vi "SWING_turn_left.vi"() -> ()   [LabVIEW 2015]
uses:
  <vilib>/NXT/Subs/MotorOutput.ctl
  <vilib>/NXT/Block Support/NXT_InputPort.ctl
  <vilib>/NXT/NXTIO Xnodes/NXTIONodeSubVIs/LEGOStopAllMotors.vi
  <vilib>/NXT/Dual Mode Library/Waits/Wait_Num.vi
  <vilib>/NXT/Dual Mode Library/Motors/MotorReverse.vi
  <vilib>/NXT/Dual Mode Library/Motors/MotorOn.vi
  <vilib>/NXT/Dual Mode Library/Sensors/Light_On.vi
  <vilib>/NXT/Dual Mode Library/Sensors/Sonar_cm.vi
  <vilib>/NXT/Dual Mode Library/Motors/MotorCoast.vi
  <vilib>/NXT/Subs/LVHSConnector.ctl
  <vilib>/NXT/NXTIO Xnodes/NXTIOXNode/NXTIO.xnode
  <vilib>/NXT/LegoClasses/BrickReference/BrickReference.lvclass
panel:
  in  "stop":bool
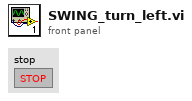
[diagram p1: front panel]
types:
  T1 = typedef "MotorOutput.ctl" = u8
  T2 = typedef "LVHSConnector.ctl" = refnum<class "BrickReference.lvclass">
  T3 = typedef "NXT_InputPort.ctl" = u32
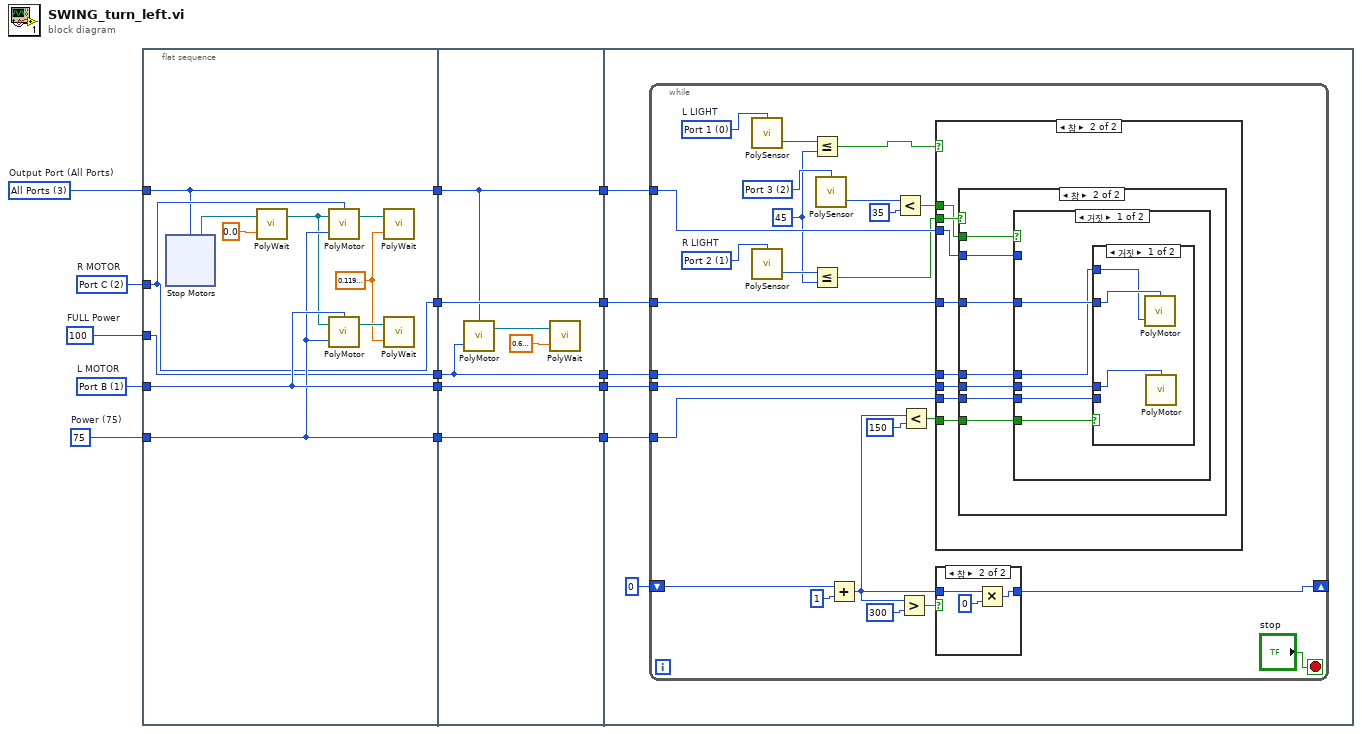
[diagram p0: block diagram]
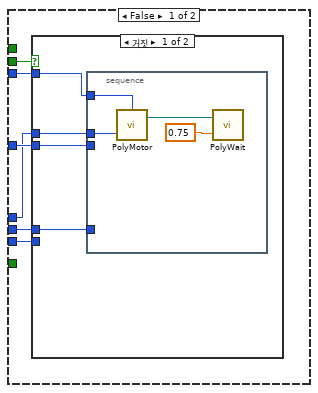
[diagram p3: hidden frame]
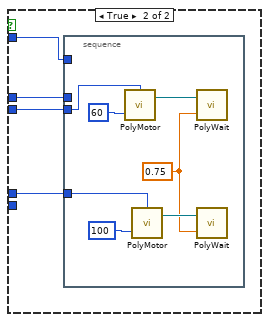
[diagram p4: hidden frame]
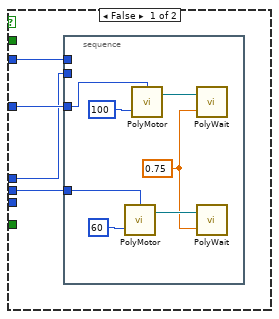
[diagram p5: hidden frame]
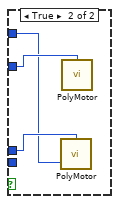
[diagram p6: hidden frame]
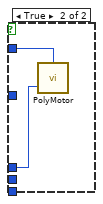
[diagram p7: hidden frame]
diagram:
  w11 = 100  # FULL Power
  w12 = 75  # Power (75)
  w13 = T1 2 items=["Port A"=0, "Port B"=1, "Port C"=2, "Ports A & B"=4, "Ports A & C"=5, "Ports B & C"=6, "All Ports"=3]  # R MOTOR
  w14 = T1 1 items=["Port A"=0, "Port B"=1, "Port C"=2, "Ports A & B"=4, "Ports A & C"=5, "Ports B & C"=6, "All Ports"=3]  # L MOTOR
  w15 = T1 3 items=["Port A"=0, "Port B"=1, "Port C"=2, "Ports A & B"=4, "Ports A & C"=5, "Ports B & C"=6, "All Ports"=3]  # Output Port (All Ports)
  n1 = flat-sequence {
    tunnel: w15 -> [w20]
    tunnel: w14 -> [w26]
    tunnel: w13 -> [w24]
    tunnel: w12 -> [w25]
    tunnel: w11 -> [w16]
    tunnel: [w20] -> w10
    tunnel: [w26] -> w8
    tunnel: [w24] -> w6
    tunnel: [w25] -> w4
    tunnel: [w16] -> w2
    tunnel: w10 -> [w34]
    tunnel: [w34] -> w9
    tunnel: w8 -> [w38]
    tunnel: [w38] -> w7
    tunnel: w6 -> [w37]
    tunnel: [w37] -> w5
    tunnel: w4 -> [w36]
    tunnel: [w36] -> w3
    tunnel: w2 -> [w35]
    tunnel: [w35] -> w1
    tunnel: w9 -> [w44]
    tunnel: w7 -> [w43]
    tunnel: w5 -> [w42]
    tunnel: w3 -> [w41]
    tunnel: w1 -> [w40]
    frame #0 {
      w21 = sgl 0.12 ("Time (1 sec)")
      n2 = xnode "Stop Motors"("Motors"=w20) -> ("NXT/EV3"=w19:T2)  [unwired: 1 in]
      n3 = call-poly <vilib>:"PolyWait.vi"("Time (1 sec)"=sgl 0.0, "NXT/EV3"=w19) -> ("NXT/EV3"=w18:T2)  [unwired: 2 in]
      n4 = call-poly <vilib>:"PolyMotor.vi"("Power (75)"=w25, "NXT/EV3"=w18, "Output Port (All Ports)"=w24) -> ("NXT/EV3"=w22:T2)  [unwired: 1 out]
      n5 = call-poly <vilib>:"PolyMotor.vi"("Power (75)"=w25, "NXT/EV3"=w18, "Output Port (All Ports)"=w26) -> ("NXT/EV3"=w23:T2)  [unwired: 1 out]
      n6 = call-poly <vilib>:"PolyWait.vi"("Time (1 sec)"=w21, "NXT/EV3"=w22) -> ()  [unwired: 2 in, 1 out]
      n7 = call-poly <vilib>:"PolyWait.vi"("Time (1 sec)"=w21, "NXT/EV3"=w23) -> ()  [unwired: 2 in, 1 out]
    }
    frame #1 {
      n8 = call-poly <vilib>:"PolyMotor.vi"("Power (75)"=w35, "Output Port (All Ports)"=w34) -> ("NXT/EV3"=w33:T2)  [unwired: 1 in, 1 out]
      n9 = call-poly <vilib>:"PolyWait.vi"("Time (1 sec)"=sgl 0.7, "NXT/EV3"=w33) -> ()  [unwired: 2 in, 1 out]
    }
    frame #2 {
      n10 = while {
        tunnel: w44 -> [w64]
        tunnel: w43 -> [w63]
        tunnel: w42 -> [w62]
        tunnel: w41 -> [w61]
        tunnel: w40 -> [w60]
        shift-right: [w50] -> _
        shift-left: i16 0 ("y") -> [w55]
        stop <- "stop" stop-if-true
        w59 = T3 2 items=["Port 1", "Port 2", "Port 3", "Port 4"] ("Port (Port 4)")
        w65 = T3 1 items=["Port 1", "Port 2", "Port 3", "Port 4"]  # R LIGHT
        w68 = T3 0 items=["Port 1", "Port 2", "Port 3", "Port 4"]  # L LIGHT
        w51 = i16 45 ("Scaled Value")
        n11 = call-poly <vilib>:"PolySensor.vi"("Port (Port 3)"=w68) -> ("Scaled Value"=w67:i16)  [unwired: 2 in, 1 out]
        n12 = call-poly <vilib>:"PolySensor.vi"("Port (Port 3)"=w65) -> ("Scaled Value"=w66:i16)  [unwired: 2 in, 1 out]
        n13 = Less Or Equal?(x=w67, y=w51) -> (x <= y?=w46:bool)
        n14 = Less Or Equal?(x=w66, y=w51) -> (x <= y?=w45:bool)
        n15 = call-poly <vilib>:"PolySensor.vi"("Port (Port 4)"=w59) -> ("Distance (cm)"=w58:i16)  [unwired: 2 in, 1 out]
        n16 = Add(x=w55, y=i16 1) -> (x+y=w49:i16)
        n17 = Less?(x=w58, y=i16 35) -> (x < y?=w56:bool)
        n18 = Greater?(x=w49, y=i16 300) -> (0:w54:bool)
        n19 = Less?(x=w49, y=i16 150) -> (x < y?=w47:bool)
        n20 = case shown="참" w46 {
          tunnel: w64 -> [w78 w106]
          tunnel: w61 -> [w77 w105]
          tunnel: w45 -> [w79 w101]
          tunnel: w62 -> [w76 w103]
          tunnel: w63 -> [w75 w104]
          tunnel: w60 -> [w74 w102]
          tunnel: w56 -> [_ w100]
          tunnel: w47 -> [_ w99]
          frame False {
            n21 = case shown="거짓" w79 {
              tunnel: w78 -> [w83 w88]
              tunnel: w77 -> [_ _]
              tunnel: w75 -> [w81 w91]
              tunnel: w76 -> [w80 w90]
              tunnel: w74 -> [w82 w89]
              frame False {
                n22 = stacked-sequence {
                  tunnel: w83 -> [w87]
                  tunnel: w82 -> [w84]
                  tunnel: w81 -> [_]
                  tunnel: w80 -> [_]
                  frame #0 {
                    n23 = call-poly <vilib>:"PolyMotor.vi"("Power (75)"=w84, "Output Port (All Ports)"=w87) -> ("NXT/EV3"=w86:T2)  [unwired: 1 in, 1 out]
                    n24 = call-poly <vilib>:"PolyWait.vi"("Time (1 sec)"=sgl 0.75, "NXT/EV3"=w86) -> ()  [unwired: 2 in, 1 out]
                  }
                }
              }
              frame True {
                n25 = stacked-sequence {
                  tunnel: w91 -> [w94]
                  tunnel: w90 -> [w93]
                  tunnel: w89 -> [_]
                  tunnel: w88 -> [_]
                  frame #0 {
                    w92 = sgl 0.75 ("Time (1 sec)")
                    n26 = call-poly <vilib>:"PolyMotor.vi"("Power (75)"=60 ("Power (75) 5"), "Output Port (All Ports)"=w93) -> ("NXT/EV3"=w95:T2)  [unwired: 1 in, 1 out]
                    n27 = call-poly <vilib>:"PolyMotor.vi"("Power (75)"=100 ("Power (75) 4"), "Output Port (All Ports)"=w94) -> ("NXT/EV3"=w96:T2)  [unwired: 1 in, 1 out]
                    n28 = call-poly <vilib>:"PolyWait.vi"("Time (1 sec)"=w92, "NXT/EV3"=w95) -> ()  [unwired: 2 in, 1 out]
                    n29 = call-poly <vilib>:"PolyWait.vi"("Time (1 sec)"=w92, "NXT/EV3"=w96) -> ()  [unwired: 2 in, 1 out]
                  }
                }
              }
            }
          }
          frame True {
            n30 = case shown="참" w101 {
              tunnel: w106 -> [w108 w124]
              tunnel: w105 -> [_ w121]
              tunnel: w104 -> [w110 w120]
              tunnel: w103 -> [w109 w119]
              tunnel: w102 -> [w107 w123]
              tunnel: w100 -> [_ w122]
              tunnel: w99 -> [_ w118]
              frame False {
                n31 = stacked-sequence {
                  tunnel: w110 -> [w115]
                  tunnel: w109 -> [w111]
                  tunnel: w108 -> [_]
                  tunnel: w107 -> [_]
                  frame #0 {
                    w112 = sgl 0.75 ("Time (1 sec)")
                    n32 = call-poly <vilib>:"PolyMotor.vi"("Power (75)"=60 ("Power (75) 2"), "Output Port (All Ports)"=w115) -> ("NXT/EV3"=w113:T2)  [unwired: 1 in, 1 out]
                    n33 = call-poly <vilib>:"PolyMotor.vi"("Power (75)"=100 ("Power (75) 3"), "Output Port (All Ports)"=w111) -> ("NXT/EV3"=w116:T2)  [unwired: 1 in, 1 out]
                    n34 = call-poly <vilib>:"PolyWait.vi"("Time (1 sec)"=w112, "NXT/EV3"=w116) -> ()  [unwired: 2 in, 1 out]
                    n35 = call-poly <vilib>:"PolyWait.vi"("Time (1 sec)"=w112, "NXT/EV3"=w113) -> ()  [unwired: 2 in, 1 out]
                  }
                }
              }
              frame True {
                n36 = case shown="거짓" w122 {
                  tunnel: w124 -> [_ w137]
                  tunnel: w123 -> [w125 w136]
                  tunnel: w121 -> [w129 _]
                  tunnel: w120 -> [w128 _]
                  tunnel: w119 -> [w127 _]
                  tunnel: w118 -> [w126 _]
                  frame False {
                    n37 = case shown="거짓" w126 {
                      tunnel: w129 -> [_ _]
                      tunnel: w128 -> [w132 w135]
                      tunnel: w127 -> [w131 w134]
                      tunnel: w125 -> [w130 w133]
                      frame False {
                        n38 = call-poly <vilib>:"PolyMotor.vi"("Power (75)"=w130, "Output Port (All Ports)"=w131) -> ()  [unwired: 1 in, 2 out]
                        n39 = call-poly <vilib>:"PolyMotor.vi"("Port (All Ports)"=w132) -> ()  [unwired: 1 in, 3 out]
                      }
                      frame True {
                        n40 = call-poly <vilib>:"PolyMotor.vi"("Power (75)"=w133, "Output Port (All Ports)"=w135) -> ()  [unwired: 1 in, 2 out]
                        n41 = call-poly <vilib>:"PolyMotor.vi"("Port (All Ports)"=w134) -> ()  [unwired: 1 in, 3 out]
                      }
                    }
                  }
                  frame True {
                    n42 = call-poly <vilib>:"PolyMotor.vi"("Power (75)"=w136, "Output Port (All Ports)"=w137) -> ()  [unwired: 1 in, 2 out]
                  }
                }
              }
            }
          }
        }
        n43 = case shown="참" w54 {
          tunnel: w49 -> [w70 w73]
          tunnel: [w70 w71] -> w50
          frame False {
          }
          frame True {
            n44 = Multiply(x=w73, y=i16 0) -> (x*y=w71:i16)
          }
        }
      }
    }
  }
